vi "SimpleDemo.vi"() -> ()   [LabVIEW 2011]
uses:
  C:/Users/Behavior Room/Desktop/Kinect Mouse/DepthSense/FunctionPointerProxy/FunctionPointerProxy/bin/Release/FunctionPointerProxy.dll
  FunctionPointerProxy/FunctionPointerProxy/bin/Release/FunctionPointerProxy.dll
  <vilib>/Platform/TimedLoop/XDataNode/timing_clust.ctl
  <vilib>/Platform/TimedLoop/XDataNode/nitl_modes.ctl
  <vilib>/Platform/TimedLoop/XDataNode/wakeup.ctl
  <vilib>/Platform/TimedLoop/XDataNode/XDataNode.xnode
  <userlib>/libOptrima-2-3/libOptrima-2-3.lvlib
  Program Files (x86)/SoftKinetic/OptrimaSDK/lib/libOptrima-2-3.dll
  <vilib>/Platform/TimedLoop/XDataNode/XDNodeRunTimeDep.lvlib
panel:
  out "Image 2":T1(plugin-control)
  out "Connect Callback?":i32
  out "Disconnect Callback?":i32
  out "API version":string
  out "NewFrame Callback?":i32
  in  "stop":bool
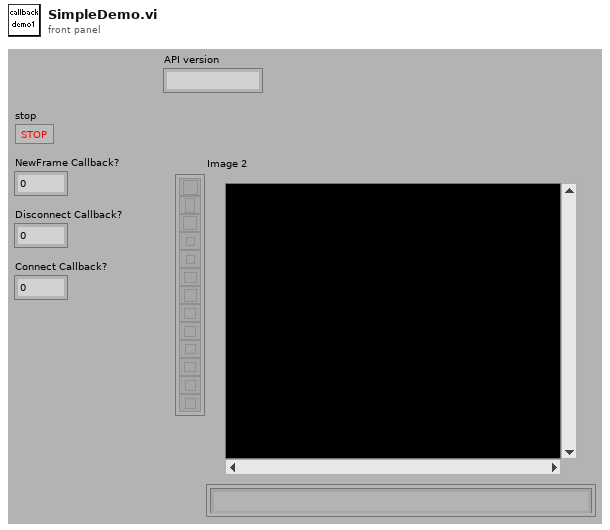
[diagram p1: front panel]
types:
  T1 = typedef "IMAQ Image.ctl" = refnum<image>
  T2 = typedef "XDNodeRunTimeDep.lvlib/timing_clust.ctl" = cluster{"Expected End [f-1]":u64, "Actual End [f-1]":u64, "Finished Late? [f-1]":bool, "Expected End [i-1]":u64, "Actual End [i-1]":u64, "Finished Late? [i-1]":bool, "Expected Start [i]":u64, "Actual Start [i]":u64, "Expected Start [f]":u64, "Actual Start [f]":u64, "Source Name":string, "Structure Name":string, "Period":i64, "Deadline":i64, "Offset":i64, "Start":i64, "Priority":i32, "Timeout":i32, "Mode":T3, "Wakeup Reason":T4, "Error":errorcluster, "Source Type":string, "Secondary Source Type":string, "Global End Time":u64, "Global Start Time":u64, "Frame Duration":u64, "Iteration Duration":u64, "Assigned CPU":i32, "I/O Scan Engine Mode":u32}
  T3 = typedef "XDNodeRunTimeDep.lvlib/nitl_modes.ctl" = enum32{"No Change", "Process missed periods, maintain original phase", "Discard missed periods, maintain original phase", "Process missed periods, ignore original phase", "Discard missed periods, ignore original phase"}
  T4 = typedef "XDNodeRunTimeDep.lvlib/wakeup.ctl" = enum32{"Normal", "Aborted", "Asynchronous wakeup", "Timing source error", "Timed loop error", "Timeout"}
  T5 = typedef "t_CallbackReferences.ctl" = cluster{"LV event callback ":refnum<k27>, "Proxy instance":refnum<k24>, "(*f)(...)":i32}
  T6 = cluster{"queue out":refnum<queue>, "queue out":refnum<queue>}
  T7 = typedef "Image Type" = u32
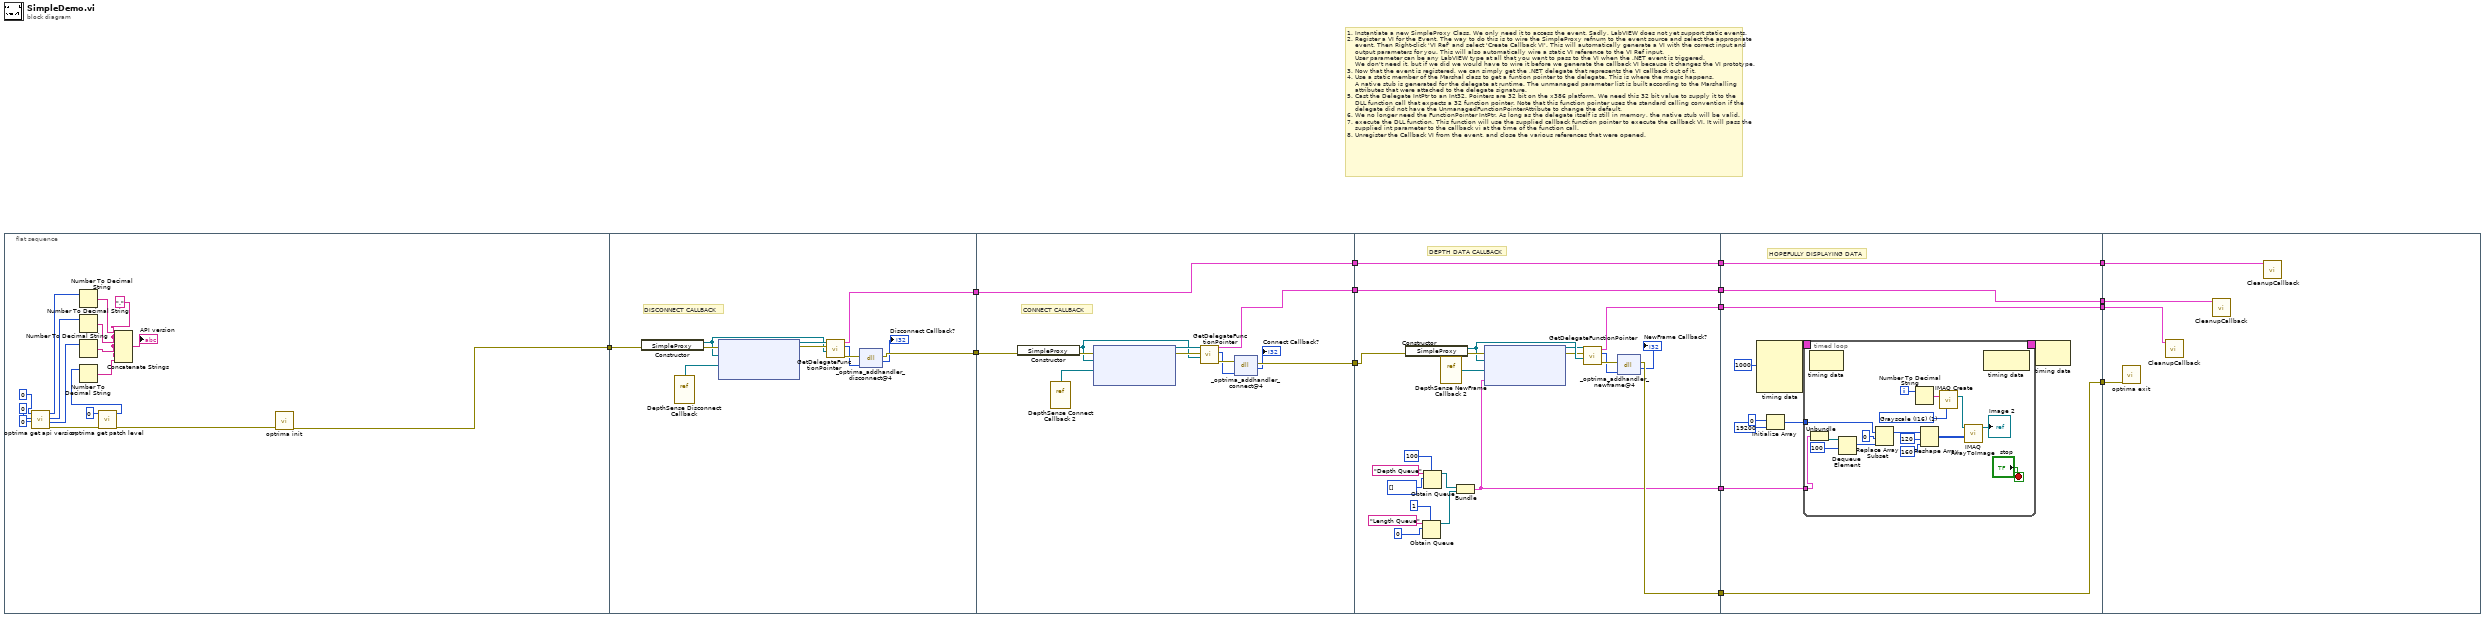
[diagram p0: block diagram]
diagram:
  # "1. Instantiate a new SimpleProxy Class. We only need it to access the event. Sadly, LabVIEW does not yet support static events.\n2. Register a VI for the Event. The way to do this is to wire the SimpleProxy refnum to the event source and select the appropriate\n    event. Then Right-click 'VI Ref' and select 'Create Callback VI'. This will automatically generate a VI with the correct input and\n    output parameters for you. This will also automatically wire a static VI reference to the VI Ref input.\n    User parameter can be any LabVIEW type at all that you want to pass to the VI when the .NET event is triggered.\n    We don't need it, but if we did we would have to wire it before we generate the callback VI because it changes the VI prototype.\n3. Now that the event is registered, we can simply get the .NET delegate that represents the VI callback out of it.\n4. Use a static member of the Marshal class to get a funtion pointer to the delegate. This is where the magic happens.\n    A native stub is generated for the delegate at runtime. The unmanaged parameter list is built according to the Marshalling\n    attributes that were attached to the delegate signature.\n5. Cast the Delegate IntPtr to an Int32. Pointers are 32 bit on the x386 platform. We need this 32 bit value to supply it to the\n    DLL function call that expects a 32 function pointer. Note that this function pointer uses the standard calling convention if the\n    delegate did not have the UnmanagedFunctionPointerAttribute to change the default.\n6. We no longer need the FunctionPointer IntPtr. As long as the delegate itself is still in memory, the native stub will be valid.\n7. execute the DLL function. This function will use the supplied callback function pointer to execute the callback VI. It will pass the\n    supplied int parameter to the callback vi at the time of the function call.\n8. Unregister the Callback VI from the event, and close the various references that were opened."
  n1 = flat-sequence {
    tunnel: [w16] -> w10
    tunnel: [w37] -> w12
    tunnel: w10 -> [w36]
    tunnel: [w33] -> w1
    tunnel: w12 -> [w48]
    tunnel: [w47] -> w11
    tunnel: [w45] -> w6
    tunnel: [w44] -> w4
    tunnel: w1 -> [w44]
    tunnel: [w77] -> w15
    tunnel: [w68] -> w14
    tunnel: w11 -> [w62]
    tunnel: [w58] -> w8
    tunnel: [w57] -> w7
    tunnel: w6 -> [w57]
    tunnel: w4 -> [w56]
    tunnel: [w56] -> w3
    tunnel: w15 -> [w87]
    tunnel: w14 -> [w88]
    tunnel: [w87] -> w13
    tunnel: [w86] -> w9
    tunnel: w8 -> [w86]
    tunnel: w7 -> [w85]
    tunnel: [w85] -> w5
    tunnel: w3 -> [w84]
    tunnel: [w84] -> w2
    tunnel: w13 -> [w114]
    tunnel: w9 -> [w113]
    tunnel: w5 -> [w112]
    tunnel: w2 -> [w111]
    frame #0 {
      w17 = "."
      n2 = call <userlib>:"optrima get api version.vi"("minor"=u32 0, "major"=u32 0, "release"=u32 0) -> ("error out"=w32:errorcluster, "minor out"=w28:u32, "major out"=w29:u32, "release out"=w30:u32)  [unwired: 5 in]
      n3 = Number To Decimal String(number=w30) -> (decimal integer string=w26:string)  [unwired: 1 in]
      n4 = Number To Decimal String(number=w29) -> (decimal integer string=w20:string)  [unwired: 1 in]
      n5 = Number To Decimal String(number=w28) -> (decimal integer string=w19:string)  [unwired: 1 in]
      n6 = call <userlib>:"optrima get patch level.vi"("error in (no error)"=w32, "patch"=u32 0) -> ("error out"=w31:errorcluster, "patch out"=w27:u32)  [unwired: 8 in]
      n7 = Number To Decimal String(number=w27) -> (decimal integer string=w18:string)  [unwired: 1 in]
      n8 = Concatenate Strings(w26, w17, w20, w17, w19, w17, w18) -> (→"API version":string)
      n9 = call <userlib>:"optrima init.vi"("error in (no error)"=w31) -> ("error out"=w16:errorcluster)  [unwired: 10 in]
    }
    frame #1 {
      # "DISCONNECT CALLBACK"
      n10 = constructor class="SimpleProxy"(error in=w36) -> (reference out=w35:refnum<k24>, error out=w43:errorcluster)  [unwired: 2 in, 1 out]
      n11 = vi-ref "DepthSense Disconnect Callback.vi"() -> ("vi reference"=w42:refnum<vi>)
      n12 = node(w43, w35, w42) -> (w41:refnum<k27>, w40:errorcluster)  [unwired: 2 in]
      n13 = call "GetDelegateFunctionPointer.vi"("target class"=w35, "error in (no error)"=w40, "event callback refnum"=w41) -> ("error out"=w39:errorcluster, "(*f)(...)"=w38:i32, "References"=w33:T5)  [unwired: 6 in]
      n14 = dll-call lib="C:/Program Files (x86)/SoftKinetic/OptrimaSDK/lib/libOptrima-2-3.dll" fn="_optrima_addhandler_disconnect@4"(error in=w39, "handlerfunc"=w38) -> (error out=w37:errorcluster, "return type"=→"Disconnect Callback?":i32)  [unwired: 3 in, 1 out]
    }
    frame #2 {
      # "CONNECT CALLBACK"
      n15 = constructor class="SimpleProxy"(error in=w48) -> (reference out=w51:refnum<k24>, error out=w55:errorcluster)  [unwired: 2 in, 1 out]
      n16 = vi-ref "DepthSense Connect Callback 2.vi"() -> ("vi reference"=w54:refnum<vi>)
      n17 = node(w55, w51, w54) -> (w53:refnum<k27>, w52:errorcluster)  [unwired: 2 in]
      n18 = call "GetDelegateFunctionPointer.vi"("target class"=w51, "error in (no error)"=w52, "event callback refnum"=w53) -> ("error out"=w50:errorcluster, "(*f)(...)"=w49:i32, "References"=w45:T5)  [unwired: 6 in]
      n19 = dll-call lib="C:/Program Files (x86)/SoftKinetic/OptrimaSDK/lib/libOptrima-2-3.dll" fn="_optrima_addhandler_connect@4"(error in=w50, "handlerfunc"=w49) -> (error out=w47:errorcluster, "return type"=→"Connect Callback?":i32)  [unwired: 3 in, 1 out]
    }
    frame #3 {
      # "DEPTH DATA CALLBACK"
      n20 = constructor class="SimpleProxy"(error in=w62) -> (reference out=w67:refnum<k24>, error out=w76:errorcluster)  [unwired: 2 in, 1 out]
      n21 = Obtain Queue(max queue size (-1, unlimited)=1, name (unnamed)="Length Queue", element data type=0) -> (queue out=w69:refnum<queue>)  [unwired: 2 in, 2 out]
      n22 = Obtain Queue(max queue size (-1, unlimited)=100, name (unnamed)="Depth Queue", element data type=u16[] [] ("p_depthmap in")) -> (queue out=w73:refnum<queue>)  [unwired: 2 in, 2 out]
      n23 = vi-ref "DepthSense NewFrame Callback 2.vi"() -> ("vi reference"=w60:refnum<vi>)
      n24 = Bundle("queue out"=w73, "queue out"=w69) -> (w68:T6)  [unwired: 1 in]
      n25 = node(w76, w67, w60, w68) -> (w65:refnum<k27>, w66:errorcluster)  [unwired: 1 in]
      n26 = call "GetDelegateFunctionPointer.vi"("target class"=w67, "error in (no error)"=w66, "event callback refnum"=w65) -> ("error out"=w64:errorcluster, "(*f)(...)"=w63:i32, "References"=w58:T5)  [unwired: 6 in]
      n27 = dll-call lib="C:/Program Files (x86)/SoftKinetic/OptrimaSDK/lib/libOptrima-2-3.dll" fn="_optrima_addhandler_newframe@4"(error in=w64, "handlerfunc"=w63) -> (error out=w77:errorcluster, "return type"=→"NewFrame Callback?":i32)  [unwired: 3 in, 1 out]
    }
    frame #4 {
      # "HOPEFULLY DISPLAYING DATA"
      n28 = node-c288(i64 1000 ("Period")) -> (w83:T2)  [unwired: 3 in]
      n29 = Initialize Array(i16 0 ("element"), 19200 ("dimension size")) -> (w78:i16[])
      n30 = timed-loop {
        tunnel: w88 -> [w103]
        timing: w83 -> [_]
        timing-out: [_] -> w82
        tunnel: w78 -> [w93]
        i -> [w100]
        stop <- "stop" stop-if-true
        w98 = T7 1 items=["Grayscale (U8)", "Grayscale (I16)", "Grayscale (SGL)", "Complex (CSG)", "RGB (U32)", "HSL (U32)", "RGB (U64)", "Grayscale (U16)"] ("Image Type")
        n31 = node-c288() -> ()  [unwired: 1 in, 1 out]
        n32 = Unbundle(w103) -> ("queue out"=w101:refnum<queue>)  [unwired: 1 out]
        n33 = Dequeue Element(queue=w101, timeout in ms (-1)=100) -> (element=w90:u16[])  [unwired: 1 in, 3 out]
        n34 = Replace Array Subset(array=w93, new element=w90, index=0) -> (w89:i16[])
        n35 = Number To Decimal String(number=w100) -> (decimal integer string=w99:string)  [unwired: 1 in]
        n36 = Reshape Array(w89, 120 ("dimension size"), 160 ("dimension size")) -> (w97:i16[][])
        n37 = call "IMAQ Create"("Image Name"=w99, "Image Type"=w98) -> ("New Image"=w94:T1)  [unwired: 3 in, 1 out]
        n38 = call "IMAQ ArrayToImage"("Image Pixels (I16)"=w97, "Image"=w94) -> ("Image Out"=→"Image 2":T1)  [unwired: 8 in, 1 out]
        n39 = node-c288() -> ()  [unwired: 1 in, 1 out]
      }
      n40 = node-c288(w82) -> ()  [unwired: 1 out]
    }
    frame #5 {
      n41 = call <userlib>:"optrima exit.vi"("error in (no error)"=w114) -> ()  [unwired: 10 in, 1 out]
      n42 = call "CleanupCallback.vi"("References"=w113) -> ()  [unwired: 10 in, 1 out]
      n43 = call "CleanupCallback.vi"("References"=w112) -> ()  [unwired: 10 in, 1 out]
      n44 = call "CleanupCallback.vi"("References"=w111) -> ()  [unwired: 10 in, 1 out]
    }
  }
